vi "Configuration File to Runtime Cluster.vi"(8 "error in (no error)":errorcluster, 11 "dsf configuration file path":path) -> (0 "error out":errorcluster, 3 "runtime configuration":T1)   [LabVIEW 2017]
uses:
  Configuration Session.lvclass
  DSF Configuration API/Public/Controls/DSF Timing Info.ctl
  DSF Configuration.lvlib
  DSF Configuration API/Public/Controls/DSF Direction.ctl
  DSF Configuration API/Public/Controls/DSF Byte Order.ctl
  DSF Configuration API/Public/Controls/DSF Data Type.ctl
  DSF Configuration API/Public/Controls/DSF Settings Info.ctl
  DSF Configuration API/Public/Controls/DSF Engine Channel Configuration.ctl
  DSF Configuration API/Public/Controls/DSF Engine Transfer Configuration.ctl
  DSF Configuration API/Public/Controls/DSF Engine Transfer Group Configuration.ctl
  DSF Configuration API/Public/Controls/DSF Engine Plugin Configuration.ctl
  DSF Configuration API/Public/Controls/DSF Engine Framework Configuration.ctl
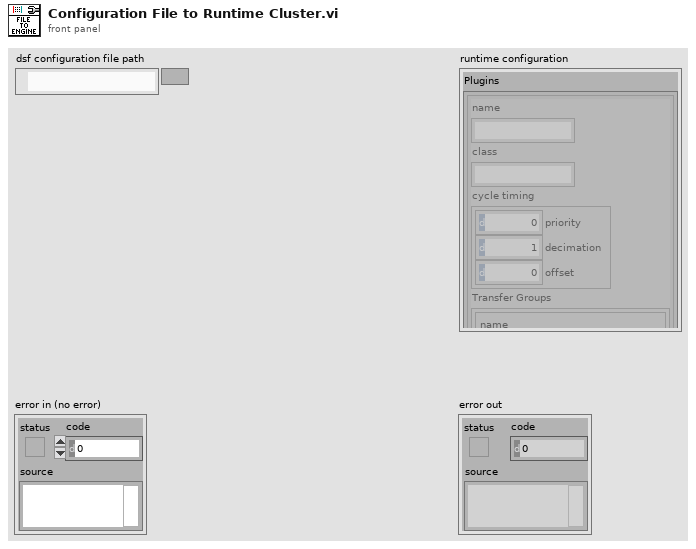
[diagram p1: front panel]
types:
  T1 = typedef "DSF Configuration.lvlib/DSF Engine Framework Configuration.ctl" = cluster{"Plugins":T2[]}
  T2 = typedef "DSF Configuration.lvlib/DSF Engine Plugin Configuration.ctl" = cluster{"name":string, "class":string, "cycle timing":T3, "Transfer Groups":T4[], "settings":T10}
  T3 = typedef "DSF Configuration.lvlib/DSF Timing Info.ctl" = cluster{"priority":u64, "decimation":u64, "offset":u64}
  T4 = typedef "DSF Configuration.lvlib/DSF Engine Transfer Group Configuration.ctl" = cluster{"name":string, "direction":T5, "cycle timing":T3, "Transfers":T6[], "settings":T10}
  T5 = typedef "DSF Configuration.lvlib/DSF Direction.ctl" = enum8{"Tx", "Rx"}
  T6 = typedef "DSF Configuration.lvlib/DSF Engine Transfer Configuration.ctl" = cluster{"name":string, "byte order":T7, "channel configurations":T8[], "settings":T10}
  T7 = typedef "DSF Configuration.lvlib/DSF Byte Order.ctl" = enum8{"big-endian", "little-endian"}
  T8 = typedef "DSF Configuration.lvlib/DSF Engine Channel Configuration.ctl" = cluster{"engine offset":u64, "name":string, "data type":T9, "count":u64, "buffer offset":u64, "settings":T10}
  T9 = typedef "DSF Configuration.lvlib/DSF Data Type.ctl" = enum8{"Bool", "SGL", "DBL", "I8", "I16", "I32", "I64", "U8", "U16", "U32", "U64"}
  T10 = typedef "DSF Configuration.lvlib/DSF Settings Info.ctl" = cluster{"key":string, "value":string}[]
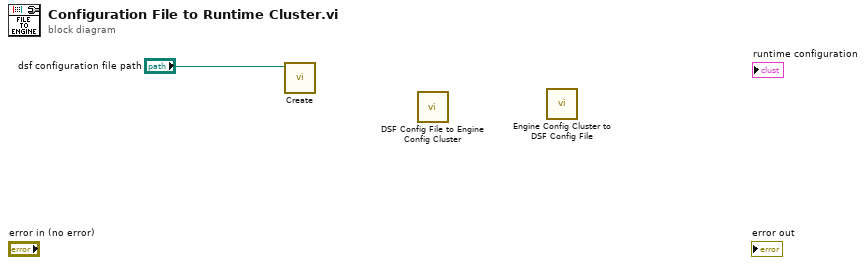
[diagram p0: block diagram]
diagram:
  n1 = call "Create.vi"("dsf configuration file path"="dsf configuration file path") -> ()  [unwired: 6 in, 5 out]
  n2 = call "DSF Config File to Engine Config Cluster.vi"() -> ()  [unwired: 10 in, 2 out]
  n3 = call "Engine Config Cluster to DSF Config File.vi"() -> ()  [unwired: 11 in, 1 out]
